vi "Get_data.vi"() -> (0 "EOF? and Error status":bool, 6 "Block Header":string)   [LabVIEW 2015]
uses:
  Controls/Block_start_and_end.ctl
  Globals/Meas_global.vi
  Globals/Trav_pos_global.vi
  Globals/LDA_meas_global_1.vi
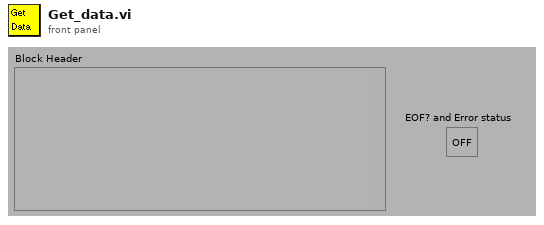
[diagram p1: front panel]
types:
  T1 = typedef "Block_start_and_end.ctl" = cluster{"Started":dbl, "Ended":dbl, "Analogue Frequency Hz":dbl}
  T2 = typedef "Post_Process.ctl" = enum16{"Take New Data", "Post Process Raw Data File"}
  T3 = typedef "PWA_Data.ctl" = enum16{"No PWA Data", "One Ch PWA"}
  T4 = typedef "BSA_Type.ctl" = enum16{"57N11", "BSA F60"}
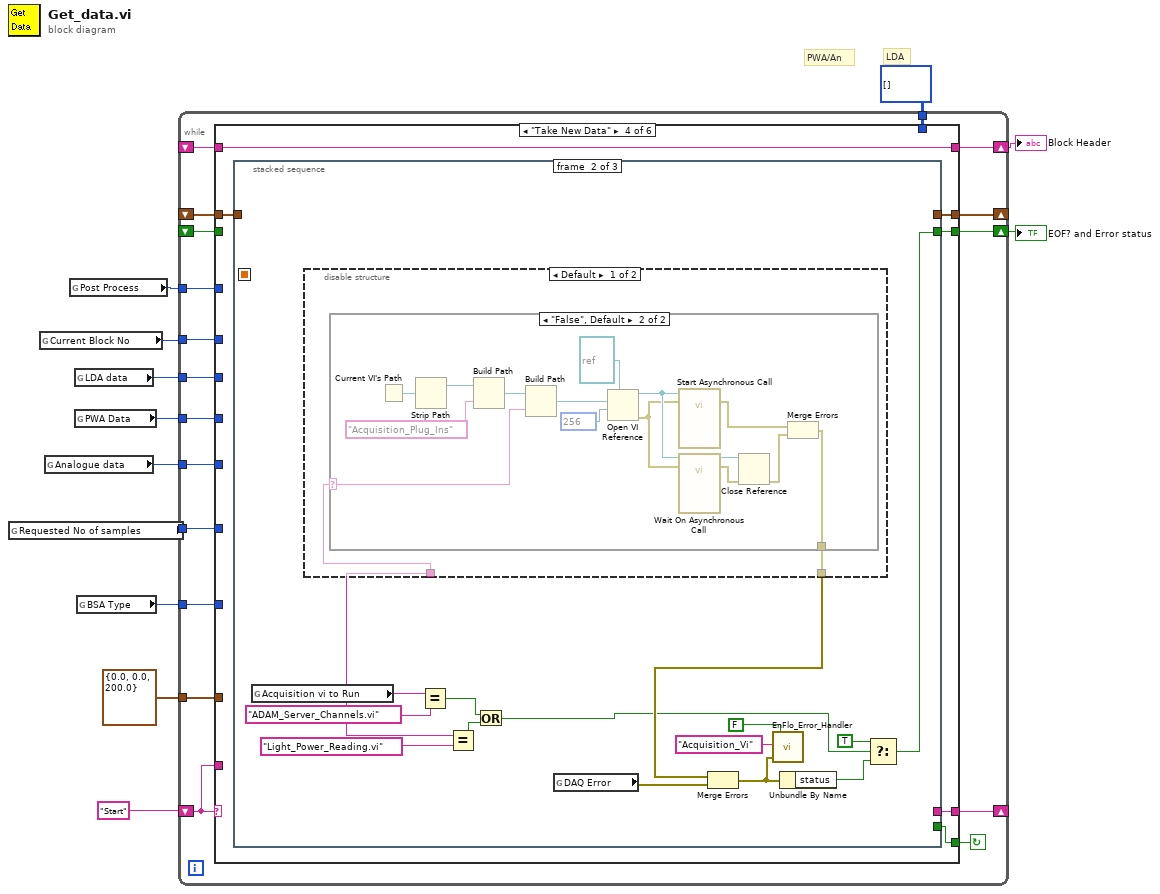
[diagram p0: block diagram]
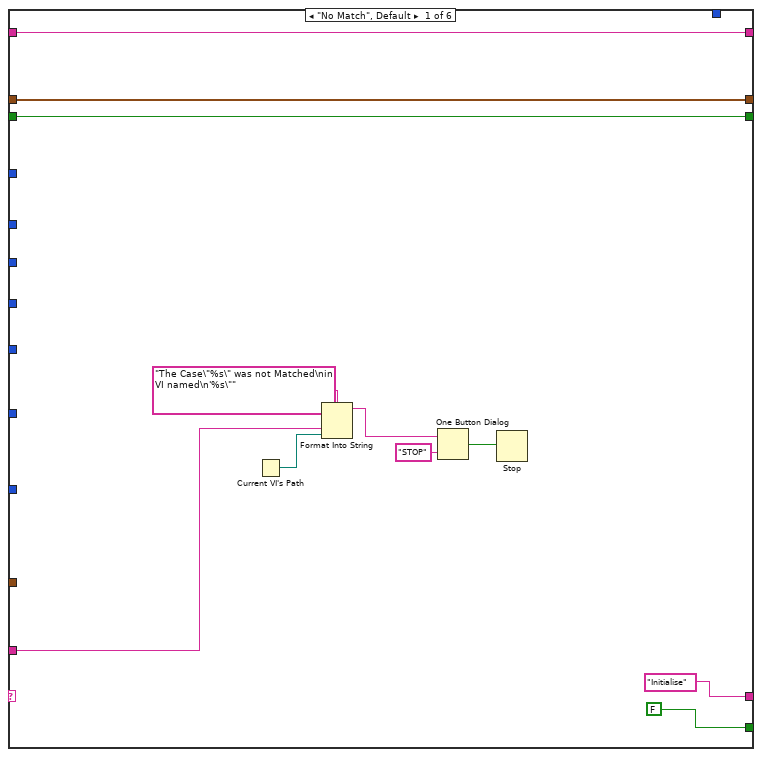
[diagram p2: hidden frame]
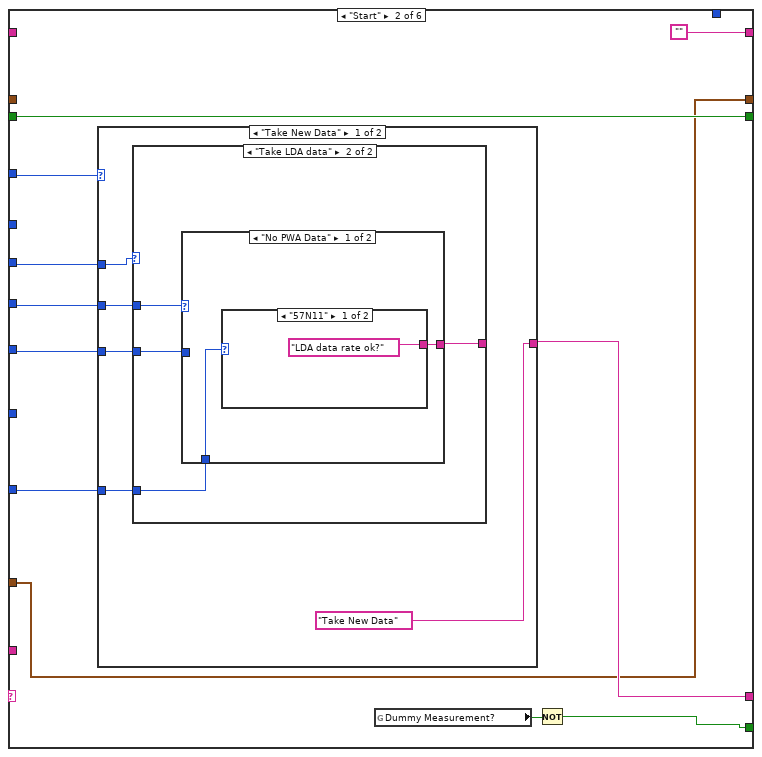
[diagram p3: hidden frame]
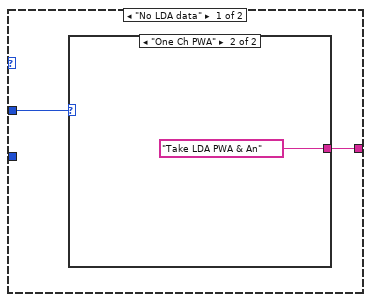
[diagram p4: hidden frame]
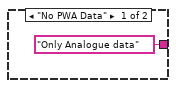
[diagram p5: hidden frame]
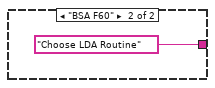
[diagram p6: hidden frame]
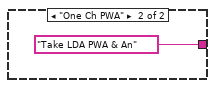
[diagram p7: hidden frame]
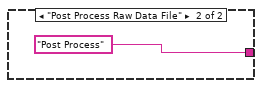
[diagram p8: hidden frame]
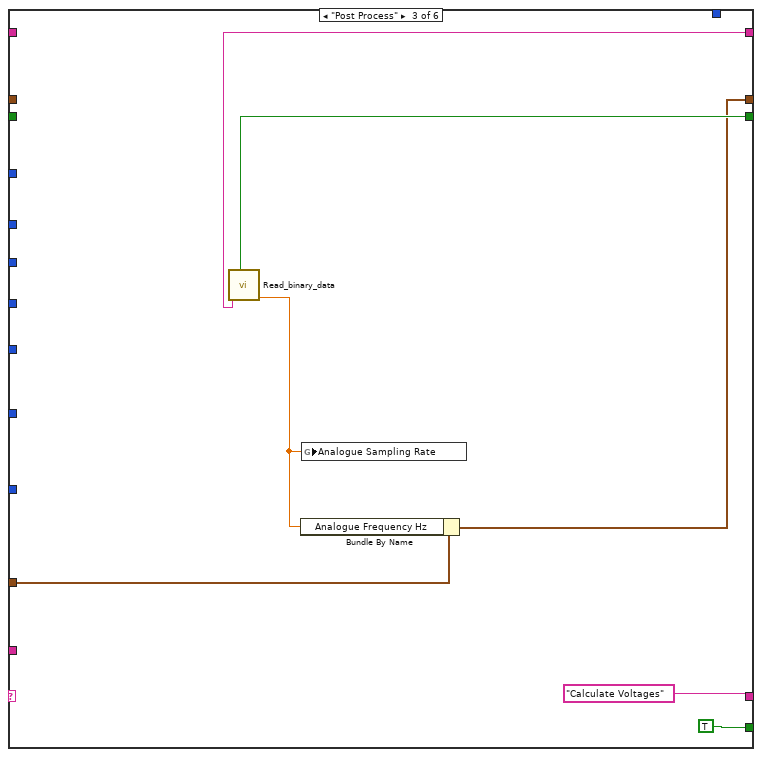
[diagram p9: hidden frame]
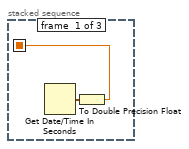
[diagram p10: hidden frame]
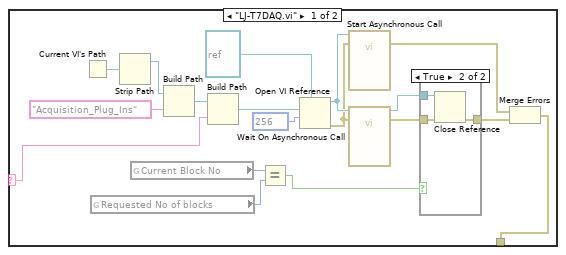
[diagram p11: hidden frame]
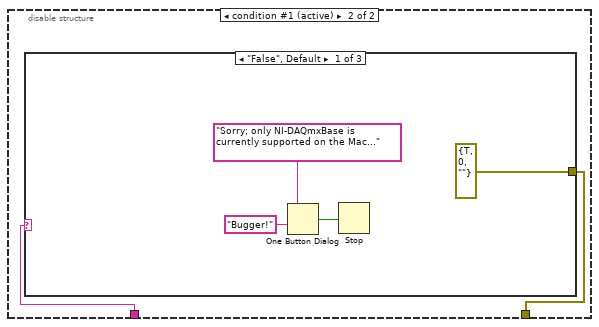
[diagram p13: hidden frame]
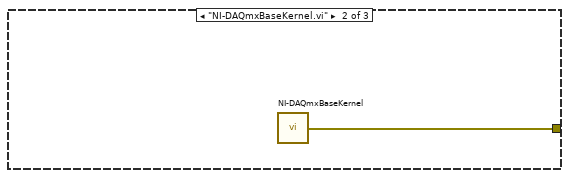
[diagram p14: hidden frame]
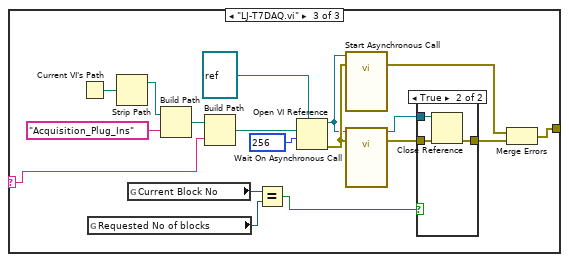
[diagram p15: hidden frame]
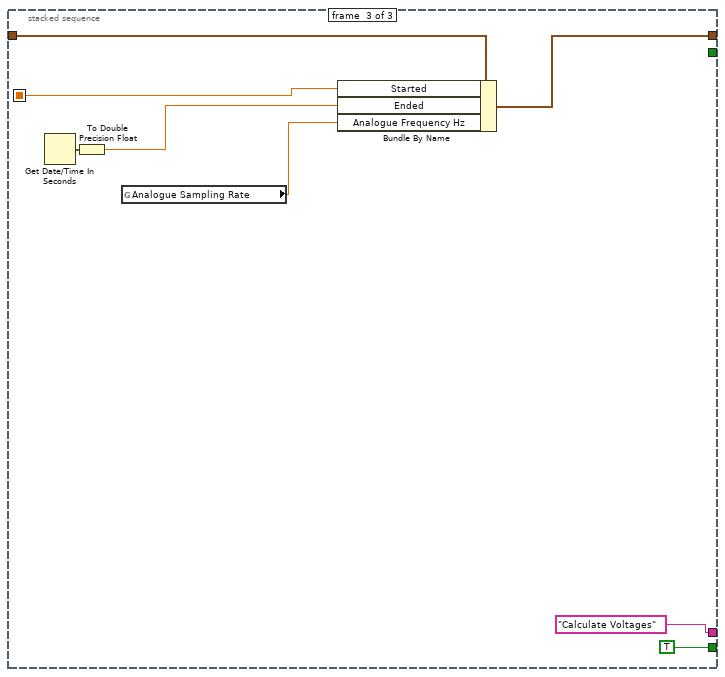
[diagram p17: hidden frame]
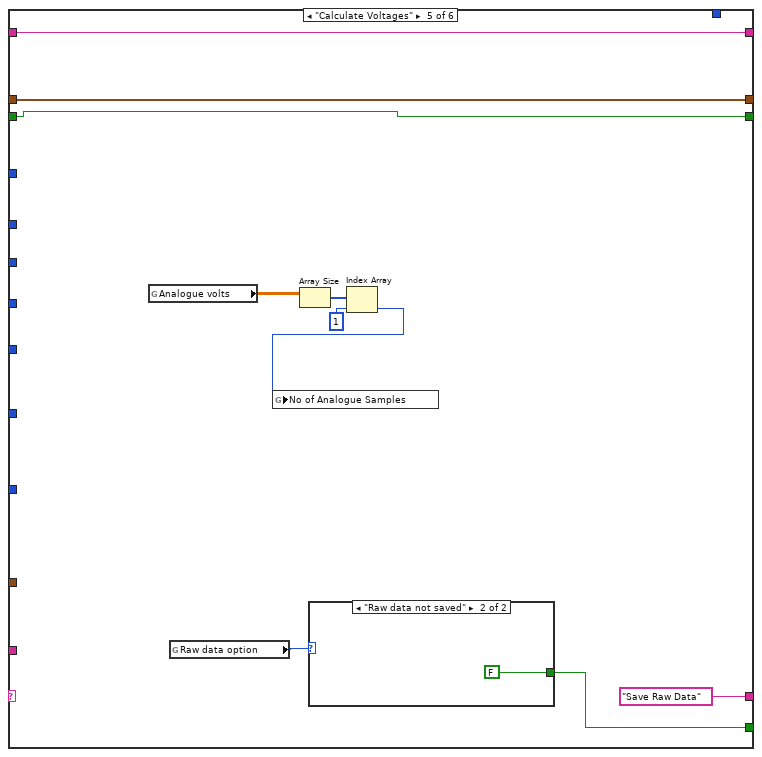
[diagram p18: hidden frame]
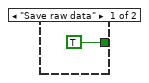
[diagram p19: hidden frame]
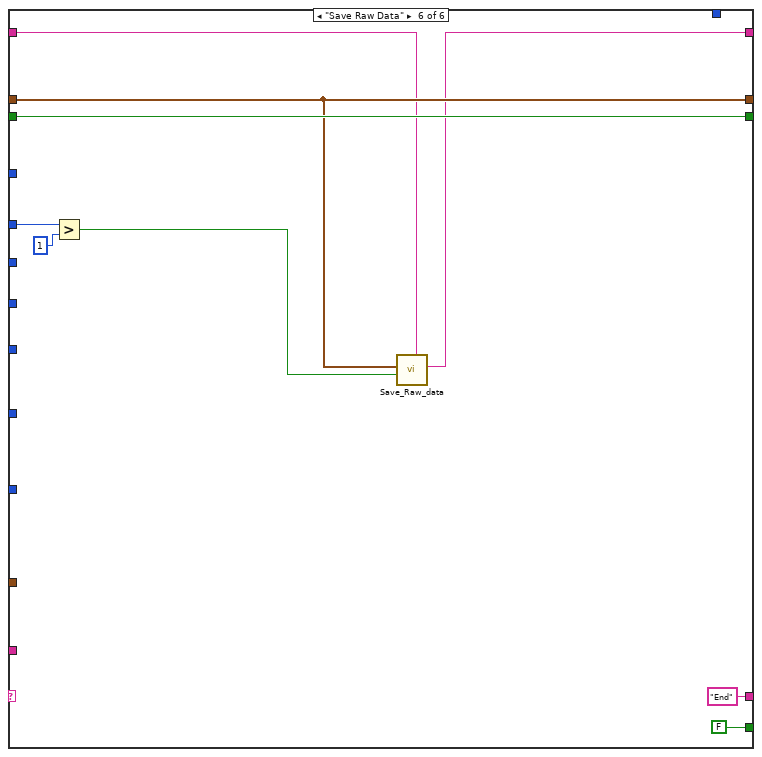
[diagram p20: hidden frame]
diagram:
  # "LDA"
  # "PWA/An"
  n1 = global read "Meas_global.vi" "Requested No of samples"() -> (w8:i32)
  n2 = global read "Meas_global.vi" "Current Block No"() -> (w7:i32)
  n3 = global read "Meas_global.vi" "Analogue data"() -> (w6:enum16{"No Analogue data", "Take Analogue data"})
  n4 = global read "Meas_global.vi" "Post Process"() -> (w9:T2)
  n5 = global read "Meas_global.vi" "LDA data"() -> (w5:enum16{"No LDA data", "Take LDA data"})
  n6 = global read "Meas_global.vi" "PWA Data"() -> (w4:T3)
  n7 = global read "LDA_meas_global_1.vi" "BSA Type"() -> (w1:T4)
  n8 = while {
    shift-left: "Start" -> [w28]
    shift-right: [w29] -> _
    shift-right: [w27] -> _
    shift-left: _ -> [w26]
    shift-right: [w25] -> w11
    shift-left: _ -> [w24]
    tunnel: T1 {"Started"=0.0, "Ended"=0.0, "Analogue Frequency Hz"=200.0} ("Block Timings") -> [w23]
    tunnel: w9 -> [w22]
    tunnel: w8 -> [w21]
    tunnel: w7 -> [w20]
    tunnel: w6 -> [w19]
    tunnel: w5 -> [w18]
    tunnel: w4 -> [w17]
    tunnel: u16[][] [] ("LDA Binary output") -> [w16]
    tunnel: w1 -> [w15]
    shift-right: [w13] -> w2
    shift-left: _ -> [w14]
    stop <- w30 continue-if-true
    n9 = case shown="\"Take New Data\"" w28 {
      tunnel: [FALSE w42 TRUE w80 w182 FALSE] -> w30
      tunnel: ["Initialise" w50 "Calculate Voltages" w81 "Save Raw Data" "End"] -> w29
      tunnel: w28 -> [w36 _ _ _ _ _]
      tunnel: [w33 w44 w74 w82 w186 w196] -> w27
      tunnel: w26 -> [w33 _ _ w83 w186 w196]
      tunnel: [w31 w52 w75 w79 w185 w197] -> w25
      tunnel: w24 -> [w31 w52 _ _ w185 w197]
      tunnel: w23 -> [_ w44 w76 _ _ _]
      tunnel: w22 -> [_ w51 _ _ _ _]
      tunnel: w21 -> [_ _ _ _ _ _]
      tunnel: w20 -> [_ _ _ _ _ w191]
      tunnel: w19 -> [_ w49 _ _ _ _]
      tunnel: w18 -> [_ w48 _ _ _ _]
      tunnel: w17 -> [_ w47 _ _ _ _]
      tunnel: w16 -> [_ _ _ _ _ _]
      tunnel: w15 -> [_ w46 _ _ _ _]
      tunnel: [w32 "" w73 w84 w181 w193] -> w13
      tunnel: w14 -> [w32 _ _ w84 w181 w192]
      frame "No Match", Default {
        n10 = Current VI's Path() -> (path=w35:path)
        n11 = Format Into String(format string="The Case\"%s\" was not Matched\nin VI named\n'%s\"" ("Format String"), w36, w35) -> (resulting string=w39:string)  [unwired: 2 in, 1 out]
        n12 = One Button Dialog(message=w39, button name ("OK")="STOP") -> (true=w37:bool)
        n13 = Stop(stop? (T)=w37) -> ()
      }
      frame "Start" {
        n14 = case shown="\"Take New Data\"" w51 {
          tunnel: ["Take New Data" "Post Process"] -> w50
          tunnel: w49 -> [w57 _]
          tunnel: w48 -> [w56 _]
          tunnel: w47 -> [w55 _]
          tunnel: w46 -> [w54 _]
          frame "Take New Data" {
            n15 = case shown="\"Take LDA data\"" w56 {
              tunnel: w57 -> [_ w63]
              tunnel: [w58 w65] -> _
              tunnel: w55 -> [w59 w64]
              tunnel: w54 -> [_ w62]
              frame "No LDA data" {
                n16 = case shown="\"One Ch PWA\"" w59 {
                  tunnel: ["Only Analogue data" "Take LDA PWA & An"] -> w58
                  frame "No PWA Data" {
                  }
                  frame "One Ch PWA" {
                  }
                }
              }
              frame "Take LDA data" {
                n17 = case shown="\"No PWA Data\"" w64 {
                  tunnel: [w66 "Take LDA PWA & An"] -> w65
                  tunnel: w63 -> [_ _]
                  tunnel: w62 -> [w67 _]
                  frame "No PWA Data" {
                    n18 = case shown="\"57N11\"" w67 {
                      tunnel: ["LDA data rate ok?" "Choose LDA Routine"] -> w66
                      frame "57N11" {
                      }
                      frame "BSA F60" {
                      }
                    }
                  }
                  frame "One Ch PWA" {
                  }
                }
              }
            }
          }
          frame "Post Process Raw Data File" {
          }
        }
        n19 = global read "Trav_pos_global.vi" "Dummy Measurement?"() -> (w43:bool)
        n20 = Not(x=w43) -> (.not. x?=w42:bool)
      }
      frame "Post Process" {
        n21 = call "Read_binary_data.vi"() -> ("Analogue Frequency Hz"=w72:dbl, "EOF?"=w75:bool, "Block Header"=w73:string)  [unwired: 7 out]
        n22 = Bundle By Name(cluster=w76, "Analogue Frequency Hz"=w72) -> (w74:T1)
        n23 = global write "Meas_global.vi" "Analogue Sampling Rate"(w72) -> ()
      }
      frame "Take New Data" {
        n24 = stacked-sequence {
          seq-local: [w85 _ _] -> [_ _ w174]
          tunnel: w83 -> [_ _ w175]
          tunnel: [_ _ w172] -> w82
          tunnel: [_ _ "Calculate Voltages"] -> w81
          tunnel: [_ _ TRUE] -> w80
          tunnel: [_ w94 _] -> w79
          frame #0 {
            n25 = Get Date/Time In Seconds() -> (seconds since 1Jan1904=w86:timestamp)
            n26 = To Double Precision Float(number=w86) -> (double precision float=w85:dbl)
          }
          frame #1 {
            n27 = global read "Meas_global.vi" "Acquisition vi to Run"() -> (w91:string)
            n28 = disable-structure shown="Default" {
              disable-tunnel: w91 -> [w101 w141]
              disable-tunnel: [w102 w140] -> w92
              frame condition #0 {
                n29 = case shown="\"False\", Default" w101 {
                  selector: w101 -> [w104 w125]
                  tunnel: [w103 w126] -> w102
                  frame "LJ-T7DAQ.vi" {
                    n30 = Current VI's Path() -> (path=w117:path)
                    n31 = global read "Meas_global.vi" "Requested No of blocks"() -> (w118:i32)
                    n32 = Strip Path(path=w117) -> (stripped path=w115:path)  [unwired: 1 out]
                    n33 = global read "Meas_global.vi" "Current Block No"() -> (w119:i32)
                    n34 = Build Path(base path=w115, name or relative path="Acquisition_Plug_Ins") -> (appended path=w114:path)
                    n35 = Build Path(base path=w114, name or relative path=w104) -> (appended path=w113:path)
                    n36 = Equal?(x=w119, y=w118) -> (x = y?=w120:bool)
                    n37 = Open VI Reference(type specifier VI Refnum (for type only)=refnum<vi> refnum, vi path=w113, options=256) -> (vi reference=w111:refnum<vi>, error out=w110:errorcluster)  [unwired: 3 in]
                    n38 = call-by-ref "Start Asynchronous Call"(reference=w111, error in=w110) -> (error out=w106:errorcluster)  [unwired: 1 in, 2 out]
                    n39 = call-by-ref "Wait On Asynchronous Call"(reference=w111, error in=w110) -> (reference out=w108:refnum<vi>, error out=w107:errorcluster)  [unwired: 1 in, 1 out]
                    n40 = case shown="True" w120 {
                      tunnel: [w121 w124] -> w105
                      tunnel: w107 -> [w121 w123]
                      tunnel: w108 -> [_ w122]
                      frame False {
                      }
                      frame True {
                        n41 = Close Reference(reference=w122, error in (no error)=w123) -> (error out=w124:errorcluster)
                      }
                    }
                    n42 = Merge Errors(w106, w105) -> (w103:errorcluster)
                  }
                  frame "False", Default {
                    n43 = Current VI's Path() -> (path=w139:path)
                    n44 = Strip Path(path=w139) -> (stripped path=w137:path)  [unwired: 1 out]
                    n45 = Build Path(base path=w137, name or relative path="Acquisition_Plug_Ins") -> (appended path=w136:path)
                    n46 = Build Path(base path=w136, name or relative path=w125) -> (appended path=w135:path)
                    n47 = Open VI Reference(type specifier VI Refnum (for type only)=refnum<vi> refnum, vi path=w135, options=256) -> (vi reference=w133:refnum<vi>, error out=w132:errorcluster)  [unwired: 3 in]
                    n48 = call-by-ref "Start Asynchronous Call"(reference=w133, error in=w132) -> (error out=w128:errorcluster)  [unwired: 1 in, 2 out]
                    n49 = call-by-ref "Wait On Asynchronous Call"(reference=w133, error in=w132) -> (reference out=w130:refnum<vi>, error out=w129:errorcluster)  [unwired: 1 in, 1 out]
                    n50 = Close Reference(reference=w130, error in (no error)=w129) -> (error out=w127:errorcluster)
                    n51 = Merge Errors(w128, w127) -> (w126:errorcluster)
                  }
                }
              }
              frame condition #1 (active) {
                n52 = case shown="\"False\", Default" w141 {
                  selector: w141 -> [_ _ w150]
                  tunnel: [errorcluster {"status"=TRUE, "code"=0, "source"=""} ("Error Out") w146 w151] -> w140
                  frame "False", Default {
                    n53 = One Button Dialog(message="Sorry; only NI-DAQmxBase is currently supported on the Mac...", button name ("OK")="Bugger!") -> (true=w143:bool)
                    n54 = Stop(stop? (T)=w143) -> ()
                  }
                  frame "NI-DAQmxBaseKernel.vi" {
                    n55 = call "NI-DAQmxBaseKernel.vi"() -> ("Error Out"=w146:errorcluster)  [unwired: 1 in]
                  }
                  frame "LJ-T7DAQ.vi" {
                    n56 = Current VI's Path() -> (path=w152:path)
                    n57 = global read "Meas_global.vi" "Requested No of blocks"() -> (w149:i32)
                    n58 = Strip Path(path=w152) -> (stripped path=w154:path)  [unwired: 1 out]
                    n59 = global read "Meas_global.vi" "Current Block No"() -> (w148:i32)
                    n60 = Build Path(base path=w154, name or relative path="Acquisition_Plug_Ins") -> (appended path=w155:path)
                    n61 = Build Path(base path=w155, name or relative path=w150) -> (appended path=w156:path)
                    n62 = Equal?(x=w148, y=w149) -> (x = y?=w147:bool)
                    n63 = Open VI Reference(type specifier VI Refnum (for type only)=refnum<vi> refnum, vi path=w156, options=256) -> (vi reference=w158:refnum<vi>, error out=w159:errorcluster)  [unwired: 3 in]
                    n64 = call-by-ref "Start Asynchronous Call"(reference=w158, error in=w159) -> (error out=w163:errorcluster)  [unwired: 1 in, 2 out]
                    n65 = call-by-ref "Wait On Asynchronous Call"(reference=w158, error in=w159) -> (reference out=w161:refnum<vi>, error out=w162:errorcluster)  [unwired: 1 in, 1 out]
                    n66 = case shown="True" w147 {
                      tunnel: [w165 w168] -> w164
                      tunnel: w162 -> [w165 w167]
                      tunnel: w161 -> [_ w166]
                      frame False {
                      }
                      frame True {
                        n67 = Close Reference(reference=w166, error in (no error)=w167) -> (error out=w168:errorcluster)
                      }
                    }
                    n68 = Merge Errors(w163, w164) -> (w151:errorcluster)
                  }
                }
              }
            }
            n69 = Equal?(x=w91, y="ADAM_Server_Channels.vi" ("Acquisition vi to Run")) -> (x = y?=w88:bool)
            n70 = Equal?(x=w91, y="Light_Power_Reading.vi" ("Acquisition vi to Run")) -> (x = y?=w89:bool)
            n71 = Or(x=w88, y=w89) -> (x .or. y?=w87:bool)
            n72 = global read "Meas_global.vi" "DAQ Error"() -> (w97:errorcluster)
            n73 = Merge Errors(w92, w97) -> (w96:errorcluster)
            n74 = call "EnFlo_Error_Handler.vi"("error in (no error)"=w96, "Error Type"="Acquisition_Vi", "Dialog Box (T)"=FALSE) -> ()  [unwired: 3 out]
            n75 = Unbundle By Name(w96) -> ("status"=w95:bool)
            n76 = Select(t=TRUE, s=w87, f=w95) -> (s? t:f=w94:bool)
          }
          frame #2 {
            n77 = Get Date/Time In Seconds() -> (seconds since 1Jan1904=w176:timestamp)
            n78 = To Double Precision Float(number=w176) -> (double precision float=w173:dbl)
            n79 = global read "Meas_global.vi" "Analogue Sampling Rate"() -> (w169:dbl)
            n80 = Bundle By Name(cluster=w175, "Started"=w174, "Ended"=w173, "Analogue Frequency Hz"=w169) -> (w172:T1)
          }
        }
      }
      frame "Calculate Voltages" {
        n81 = global read "Meas_global.vi" "Analogue volts"() -> (w177:dbl[][])
        n82 = global read "Meas_global.vi" "Raw data option"() -> (w184:enum16{"Save raw data", "Raw data not saved"})
        n83 = Array Size(array=w177) -> (size(s)=w178:i32[])
        n84 = case shown="\"Raw data not saved\"" w184 {
          tunnel: [TRUE FALSE] -> w182
          frame "Save raw data" {
          }
          frame "Raw data not saved" {
          }
        }
        n85 = Index Array(array=w178, index=1) -> (element=w180:i32)
        n86 = global write "Meas_global.vi" "No of Analogue Samples"(w180) -> ()
      }
      frame "Save Raw Data" {
        n87 = Greater?(x=w191, y=1) -> (0:w189:bool)
        n88 = call "Save_Raw_data.vi"("Add to Block Header"=w192, "append to file? (new file:F)"=w189, "Block Timings"=w196) -> ("Block Header"=w193:string)  [unwired: 6 in]
      }
    }
  }
  "EOF? and Error status" <- w11
  "Block Header" <- w2
